vi "直通基准_control switch.vi"(8 "error in (no error)":errorcluster, 9 "COM":i32, 11 "A":i32) -> (0 "error out":errorcluster)   [LabVIEW 2011]
uses:
  network_Global/Global.vi
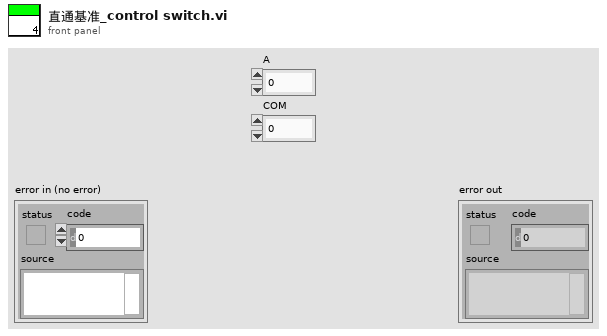
[diagram p1: front panel]
types:
  T1 = typedef "通道.ctl" = cluster{"用户名":string, "RF进口":string, "RF出口":string, "CLK进口":string, "CLK出口":string, "FCLK进口":string, "FCLK出口":string, "时间":u16}
  T2 = cluster{"用户名":string, "RF进口":string, "RF出口":string, "CLK进口":string, "CLK出口":string, "FCLK进口":string, "FCLK出口":string, "时间":u16}
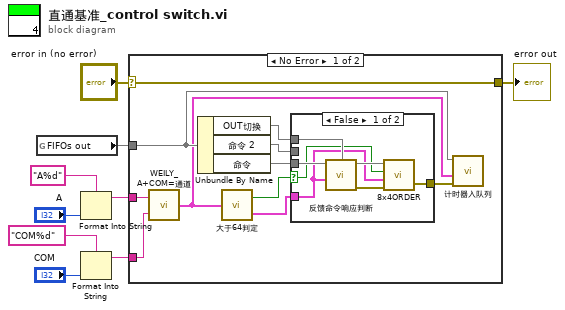
[diagram p0: block diagram]
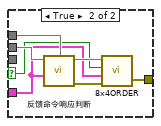
[diagram p2: hidden frame]
diagram:
  n1 = global read "Global.vi" "FIFOs out"() -> (w7)
  n2 = Format Into String(format string="A%d", "A") -> (resulting string=w2:string)  [unwired: 2 in, 1 out]
  n3 = Format Into String(format string="COM%d", "COM") -> (resulting string=w1:string)  [unwired: 2 in, 1 out]
  n4 = case shown="No Error" "error in (no error)" {
    selector: "error in (no error)" -> [w20 w33]
    tunnel: [w20 w33] -> w8
    tunnel: w7 -> [w14 _]
    tunnel: w2 -> [w11 _]
    tunnel: w1 -> [w10 _]
    frame No Error {
      n5 = call "WEILY_A+COM=通道.vi"("RF出口"=w10, "RF进口"=w11) -> ("通道"=w12:T1)
      n6 = Unbundle By Name(w14) -> ("OUT切换"=w17, "命令 2"=w16, "命令"=w15)
      n7 = call "大于64判定.vi"("通道"=w12) -> (">64"=w19:bool, "通道(出)"=w18:T2)
      n8 = case shown="False" w19 {
        selector: w19 -> [w22 w28]
        tunnel: [w24 w30] -> w13
        tunnel: w15 -> [w26 _]
        tunnel: w18 -> [w21 w27]
        tunnel: w16 -> [_ w32]
        tunnel: w17 -> [w23 w29]
        frame False {
          n9 = call "反馈命令响应判断.vi"("通道"=w21, "命令"=w26) -> ("error out"=w25:errorcluster)  [unwired: 5 in]
          n10 = call "8x4ORDER.vi"("error in"=w25, "通道"=w21, ">64"=w22, "OUT切换"=w23) -> ("error out"=w24:errorcluster)  [unwired: 1 out]
        }
        frame True {
          n11 = call "反馈命令响应判断.vi"("通道"=w27, "命令"=w32) -> ("error out"=w31:errorcluster)  [unwired: 5 in]
          n12 = call "8x4ORDER.vi"("error in"=w31, "通道"=w27, ">64"=w28, "OUT切换"=w29) -> ("error out"=w30:errorcluster)  [unwired: 1 out]
        }
      }
      n13 = call "计时器入队列.vi"("error in"=w13, "通道"=w12, "FIFOs in"=w14) -> ()  [unwired: 4 in, 1 out]
    }
    frame Error {
    }
  }
  "error out" <- w8
